vi "OpenPiezo.vi"(9 "MG17Piezo X":refnum<k7>(container), 10 "MG17Piezo Y":refnum<k7>(container), 11 "MG17Piezo Z":refnum<k7>(container)) -> (0 "error out Z":errorcluster, 1 "error out Y":errorcluster, 2 "MG17 X":refnum<k7>, 3 "MG17 Y":refnum<k7>, 4 "error out X":errorcluster, 5 "MG17 Z":refnum<k7>)   [LabVIEW 2014]
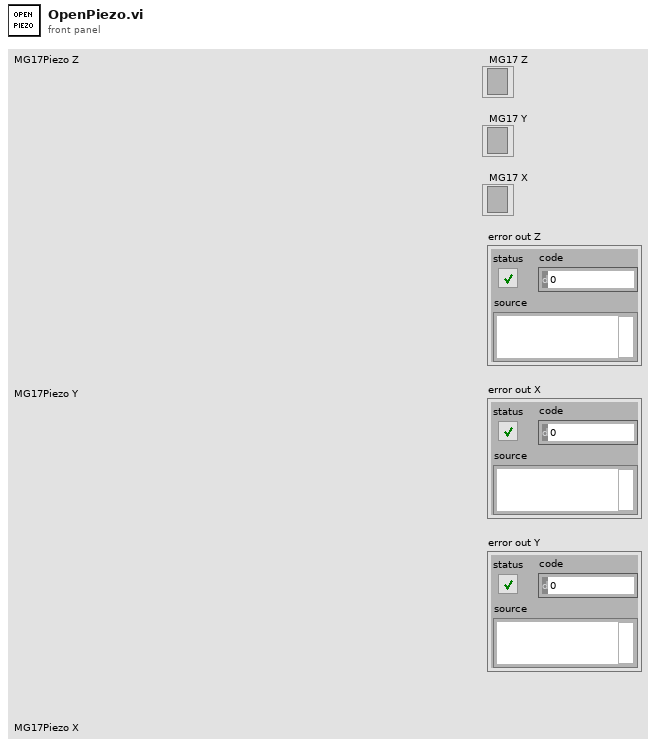
[diagram p1: front panel]
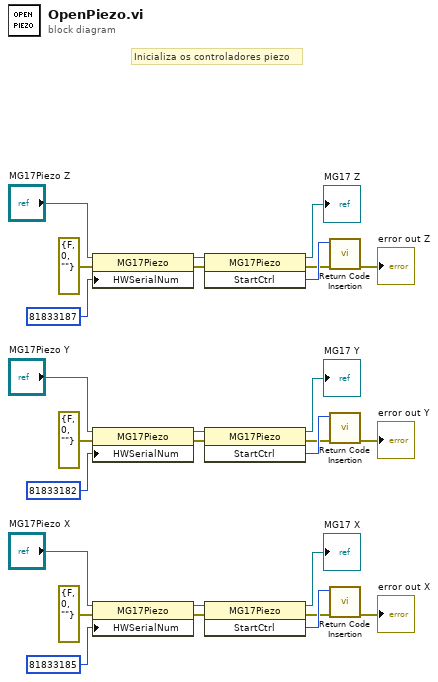
[diagram p0: block diagram]
diagram:
  # "Inicializa os controladores piezo"
  n1 = property class="MG17Piezo"(reference="MG17Piezo Z", error in=errorcluster {"status"=FALSE, "code"=0, "source"=""} ("error in (no error)"), "HWSerialNum"=81833187) -> (reference out=w2:refnum<k7>, error out=w5:errorcluster)
  n2 = property class="MG17Piezo"(reference="MG17Piezo Y", error in=errorcluster {"status"=FALSE, "code"=0, "source"=""} ("error in (no error)"), "HWSerialNum"=81833182) -> (reference out=w11:refnum<k7>, error out=w14:errorcluster)
  n3 = property class="MG17Piezo"(reference="MG17Piezo X", error in=errorcluster {"status"=FALSE, "code"=0, "source"=""} ("error in (no error)"), "HWSerialNum"=81833185) -> (reference out=w18:refnum<k7>, error out=w21:errorcluster)
  n4 = invoke class="MG17Piezo" method="StartCtrl"(reference=w2, error in=w5) -> (reference out=→"MG17 Z":refnum<k7>, error out=w6:errorcluster, "StartCtrl"=w8:i32)  [unwired: 1 in]
  n5 = invoke class="MG17Piezo" method="StartCtrl"(reference=w11, error in=w14) -> (reference out=→"MG17 Y":refnum<k7>, error out=w15:errorcluster, "StartCtrl"=w16:i32)  [unwired: 1 in]
  n6 = invoke class="MG17Piezo" method="StartCtrl"(reference=w18, error in=w21) -> (reference out=→"MG17 X":refnum<k7>, error out=w22:errorcluster, "StartCtrl"=w23:i32)  [unwired: 1 in]
  n7 = call "Return Code Insertion.vi"("error in (no error)"=w6, "Return Code"=w8) -> ("error out"=→"error out Z":errorcluster)  [unwired: 9 in]
  n8 = call "Return Code Insertion.vi"("error in (no error)"=w15, "Return Code"=w16) -> ("error out"=→"error out Y":errorcluster)  [unwired: 9 in]
  n9 = call "Return Code Insertion.vi"("error in (no error)"=w22, "Return Code"=w23) -> ("error out"=→"error out X":errorcluster)  [unwired: 9 in]
